vi "SUB-module-현재 VI 경로.vi"() -> (0 "현재 VI 경로":path)   [LabVIEW 2015]
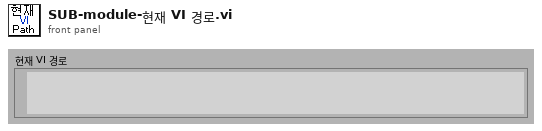
[diagram p1: front panel]
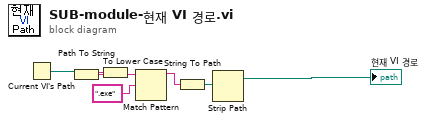
[diagram p0: block diagram]
diagram:
  n1 = Current VI's Path() -> (path=w6:path)
  n2 = Path To String(path=w6) -> (string=w5:string)
  n3 = To Lower Case(string=w5) -> (all lower case string=w3:string)
  n4 = Match Pattern(string=w3, regular expression=".exe" ("search string")) -> (before substring=w2:string)  [unwired: 4 out]
  n5 = String To Path(string=w2) -> (path=w1:path)
  n6 = Strip Path(path=w1) -> (stripped path=→"현재 VI 경로":path)  [unwired: 1 out]
